vi "Finish Round.vi"(7 "Round":u32, 9 "Teams In":refnum<class "Team.lvclass">[](array[class]), 11 "Map in":refnum<class "Map.lvclass">) -> (1 "Teams":refnum<class "Team.lvclass">[](array[class]), 3 "Map out":refnum<class "Map.lvclass">)   [LabVIEW 2020, in "SquareBattle.lvlib" / "Map.lvclass"]
uses:
  Map.lvclass
  Team/Team.lvclass
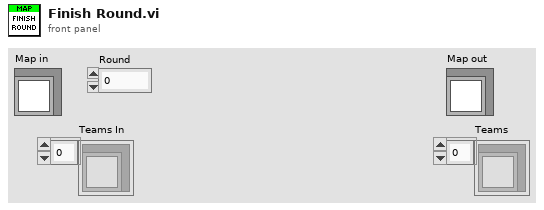
[diagram p1: front panel]
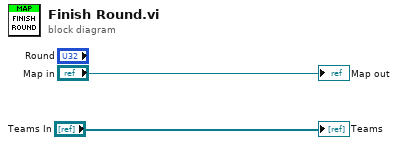
[diagram p0: block diagram]
diagram:
  "Map out" <- "Map in"
  "Teams" <- "Teams In"
